vi "Update State on Cursor Move.vi"(8 "Cursor.Position.X":dbl, 9 "Cursor Name":string, 11 "Display State In":T1={"Graph Visible Items"={"Plot Legend"=FALSE, "Scale Legend"=FALSE, "Graph Palette"=FALSE, "Cursor Legend"=FALSE, "X Scrollbar"=FALSE}, "View Table"=FALSE, "Table Visible Items"={"Vertical Scrollbar"=FALSE, "Horizontal Scrollbar"=FALSE, "Row Headers"=FALSE, "Column Headers"=FALSE, "Vertical Lines"=FALSE, "Horizontal Lines"=FALSE}, "Header Font"={"Font Name"="", "Size"=0, "Bold"=FALSE, "Italic"=FALSE, "Underline"=FALSE, "Strikeout"=FALSE, "Color"=0}, "Cell Font"={"Font Name"="", "Size"=0, "Bold"=FALSE, "Italic"=FALSE, "Underline"=FALSE, "Strikeout"=FALSE, "Color"=0}, "Description and Tip..."={"Description"="", "Tip"=""}, "Moveable Splitter Position"=0, "Measurement Cursor Configuration"={"XY"={"enable XY"=FALSE, "Position (X)"=[], "Type"=enum."Absolute", "Y reference"=0.0, "color"=0}, "band"={"enable band"=FALSE, "B1"=0.0, "B2"=0.0, "Fixed bandwidth (B2-B1)"=0.0, "B1 color"=0, "B2 color"=0}, "harmonic"={"enable harmonics"=FALSE, "X reference (1X)"=0.0, "Maximum"=0, "Subset"=enum."All", "1X color"=0, "MX color"=0}, "sideband"={"enable sideband"=FALSE, "X center (C)"=0.0, "Sidebands"=0, "X spacing (s)"=0.0, "Center color"=0, "Sideband color"=0}}, "Cursors"={"List"=[], "Tags"=[]}, "X Increment"=0.0, "X Scale"={"Label Visible"=FALSE, "Label Text"="", "Mapping Mode"=0, "Format String"=""}, "Y Scale"={"Label Visible"=FALSE, "Label Text"="", "Mapping Mode"=0, "Format String"=""}, "Colors"={"background"=16777215, "major grid"=8355711, "minor grid"=12632256, "font"=0}, "desired spectrum view"={"scaling"={"linear/dB"=enum."no change", "dB reference"=0.0, "power/magnitude"=enum."no change", "view"=enum."no change"}, "spectral density"=enum."no change"}, "Plot Color Wheel"=[3381759, 32768, 982784, 4375295, 13827953, 13457919, 16757522, 4343295, 16728758, 12095254], "Plots"=[], "registered user events"=variant, "Lock 1X to Peak"=FALSE} caption="State" {"Y Scale"."Mapping Mode" items=["Linear", "Logarithmic", "dB"]; "X Scale"."Mapping Mode" items=["Linear", "Logarithmic"]}) -> (0 "cursor type":string, 1 "cursor index":i32, 3 "Display State Out":T1={"Graph Visible Items"={"Plot Legend"=FALSE, "Scale Legend"=FALSE, "Graph Palette"=FALSE, "Cursor Legend"=FALSE, "X Scrollbar"=FALSE}, "View Table"=FALSE, "Table Visible Items"={"Vertical Scrollbar"=FALSE, "Horizontal Scrollbar"=FALSE, "Row Headers"=FALSE, "Column Headers"=FALSE, "Vertical Lines"=FALSE, "Horizontal Lines"=FALSE}, "Header Font"={"Font Name"="", "Size"=0, "Bold"=FALSE, "Italic"=FALSE, "Underline"=FALSE, "Strikeout"=FALSE, "Color"=0}, "Cell Font"={"Font Name"="", "Size"=0, "Bold"=FALSE, "Italic"=FALSE, "Underline"=FALSE, "Strikeout"=FALSE, "Color"=0}, "Description and Tip..."={"Description"="", "Tip"=""}, "Moveable Splitter Position"=0, "Measurement Cursor Configuration"={"XY"={"enable XY"=FALSE, "Position (X)"=[], "Type"=enum."Absolute", "Y reference"=0.0, "color"=0}, "band"={"enable band"=FALSE, "B1"=0.0, "B2"=0.0, "Fixed bandwidth (B2-B1)"=0.0, "B1 color"=0, "B2 color"=0}, "harmonic"={"enable harmonics"=FALSE, "X reference (1X)"=0.0, "Maximum"=0, "Subset"=enum."All", "1X color"=0, "MX color"=0}, "sideband"={"enable sideband"=FALSE, "X center (C)"=0.0, "Sidebands"=0, "X spacing (s)"=0.0, "Center color"=0, "Sideband color"=0}}, "Cursors"={"List"=[], "Tags"=[]}, "X Increment"=0.0, "X Scale"={"Label Visible"=FALSE, "Label Text"="", "Mapping Mode"=0, "Format String"=""}, "Y Scale"={"Label Visible"=FALSE, "Label Text"="", "Mapping Mode"=0, "Format String"=""}, "Colors"={"background"=16777215, "major grid"=8355711, "minor grid"=12632256, "font"=0}, "desired spectrum view"={"scaling"={"linear/dB"=enum."no change", "dB reference"=0.0, "power/magnitude"=enum."no change", "view"=enum."no change"}, "spectral density"=enum."no change"}, "Plot Color Wheel"=[3381759, 32768, 982784, 4375295, 13827953, 13457919, 16757522, 4343295, 16728758, 12095254], "Plots"=[], "registered user events"=variant, "Lock 1X to Peak"=FALSE} caption="State" {"Y Scale"."Mapping Mode" items=["Linear", "Logarithmic", "dB"]; "X Scale"."Mapping Mode" items=["Linear", "Logarithmic"]})   [LabVIEW 2017, in "Octave with Cursors.xctl"]
doc: "Within Display State, moves linked cursors in set."
uses:
  <vilib>/addons/_XControls/Octave with Cursors/Octave with Cursors.xctl
  <vilib>/addons/_XControls/Octave with Cursors/Controls/State.ctl
  <vilib>/Utility/miscctls.llb/LVFontTypeDef.ctl
  <vilib>/addons/_XControls/Octave with Cursors/Controls/Measurement Cursor Configuration.ctl
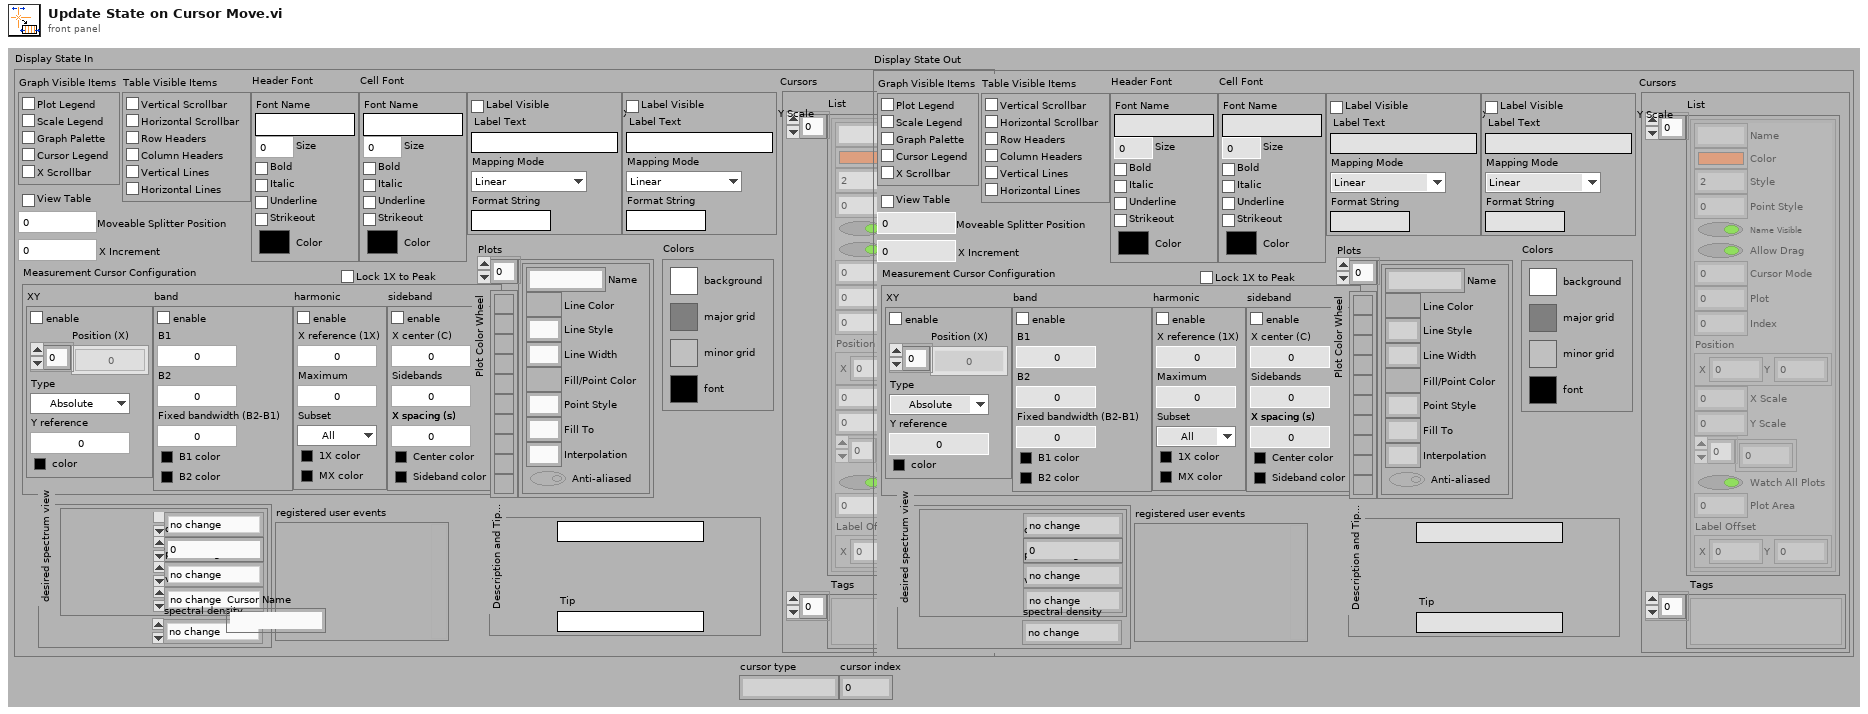
[diagram p1: front panel]
types:
  T1 = typedef "Octave with Cursors.xctl/State.ctl" = cluster{"Graph Visible Items":cluster{"Plot Legend":bool, "Scale Legend":bool, "Graph Palette":bool, "Cursor Legend":bool, "X Scrollbar":bool}, "View Table":bool, "Table Visible Items":cluster{"Vertical Scrollbar":bool, "Horizontal Scrollbar":bool, "Row Headers":bool, "Column Headers":bool, "Vertical Lines":bool, "Horizontal Lines":bool}, "Header Font":T2, "Cell Font":T2, "Description and Tip...":cluster{"Description":string, "Tip":string}, "Moveable Splitter Position":i32, "Measurement Cursor Configuration":T3, "Cursors":cluster{"List":cluster{"Name":string, "Color":u32, "Style":i32, "Point Style":u8, "Name Visible":bool, "Allow Drag":bool, "Cursor Mode":u32, "Plot":i32, "Index":i32, "Position":cluster{"X":dbl, "Y":dbl}, "X Scale":u32, "Y Scale":u32, "Watch Plots":i32[], "Watch All Plots":bool, "Plot Area":i32, "Label Offset":cluster{"X":dbl, "Y":dbl}}[], "Tags":variant[]}, "X Increment":dbl, "X Scale":cluster{"Label Visible":bool, "Label Text":string, "Mapping Mode":u8, "Format String":string}, "Y Scale":cluster{"Label Visible":bool, "Label Text":string, "Mapping Mode":u8, "Format String":string}, "Colors":cluster{"background":u32, "major grid":u32, "minor grid":u32, "font":u32}, "desired spectrum view":cluster{"scaling":cluster{"linear/dB":enum16{"no change", "linear", "dB"}, "dB reference":dbl, "power/magnitude":enum16{"no change", "power", "magnitude"}, "view":enum16{"no change", "rms", "peak", "peak-peak"}}, "spectral density":enum16{"no change", "spectrum", "spectral density"}}, "Plot Color Wheel":u32[], "Plots":cluster{"Name":string, "Line Color":u32, "Line Style":u8, "Line Width":u8, "Fill/Point Color":u32, "Point Style":u8, "Fill To":i16, "Interpolation":u8, "Anti-aliased":bool}[], "registered user events":variant, "Lock 1X to Peak":bool}
  T2 = typedef "LVFontTypeDef.ctl" = cluster{"Font Name":string, "Size":u16, "Bold":bool, "Italic":bool, "Underline":bool, "Strikeout":bool, "Color":u32}
  T3 = typedef "Octave with Cursors.xctl/Measurement Cursor Configuration.ctl" = cluster{"XY":cluster{"enable XY":bool, "Position (X)":dbl[], "Type":enum16{"Absolute", "Relative"}, "Y reference":dbl, "color":u32}, "band":cluster{"enable band":bool, "B1":dbl, "B2":dbl, "Fixed bandwidth (B2-B1)":dbl, "B1 color":u32, "B2 color":u32}, "harmonic":cluster{"enable harmonics":bool, "X reference (1X)":dbl, "Maximum":i32, "Subset":enum16{"All", "Even", "Odd"}, "1X color":u32, "MX color":u32}, "sideband":cluster{"enable sideband":bool, "X center (C)":dbl, "Sidebands":i32, "X spacing (s)":dbl, "Center color":u32, "Sideband color":u32}}
  T4 = cluster{"Name":string, "Color":u32, "Style":i32, "Point Style":u8, "Name Visible":bool, "Allow Drag":bool, "Cursor Mode":u32, "Plot":i32, "Index":i32, "Position":cluster{"X":dbl, "Y":dbl}, "X Scale":u32, "Y Scale":u32, "Watch Plots":i32[], "Watch All Plots":bool, "Plot Area":i32, "Label Offset":cluster{"X":dbl, "Y":dbl}}[]
  T5 = cluster{"Name":string, "Color":u32, "Style":i32, "Point Style":u8, "Name Visible":bool, "Allow Drag":bool, "Cursor Mode":u32, "Plot":i32, "Index":i32, "Position":cluster{"X":dbl, "Y":dbl}, "X Scale":u32, "Y Scale":u32, "Watch Plots":i32[], "Watch All Plots":bool, "Plot Area":i32, "Label Offset":cluster{"X":dbl, "Y":dbl}}
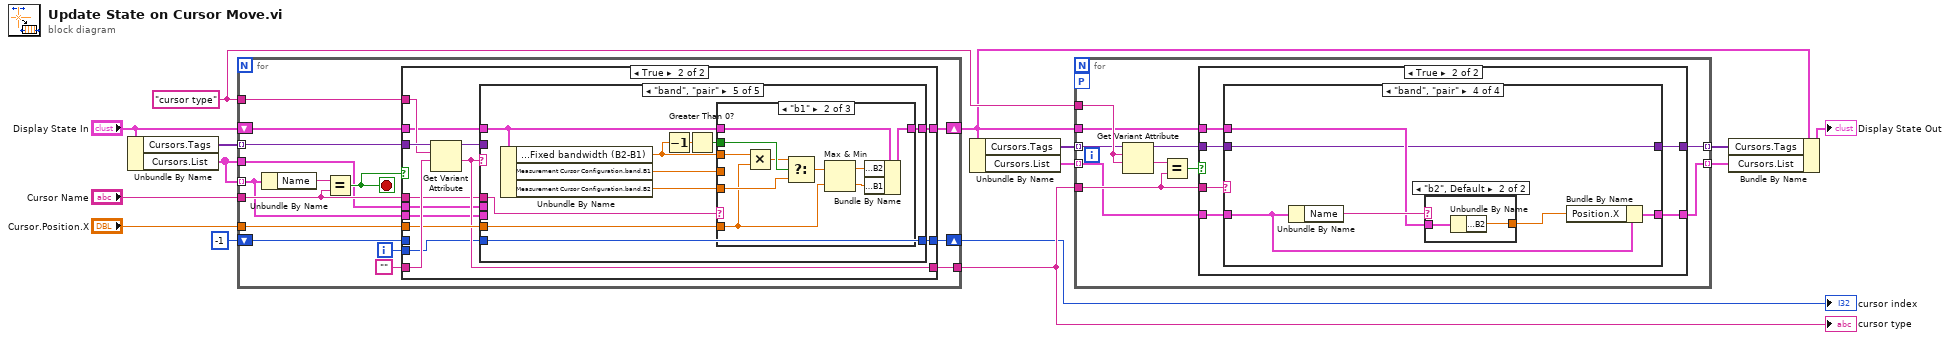
[diagram p0: block diagram]
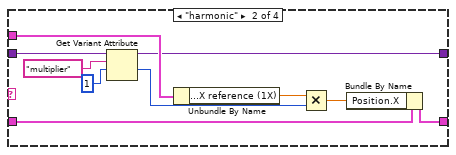
[diagram p4: hidden frame]
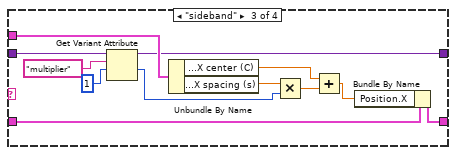
[diagram p5: hidden frame]
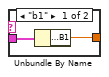
[diagram p6: hidden frame]
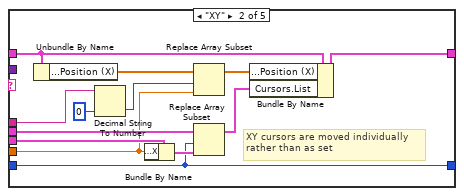
[diagram p9: hidden frame]
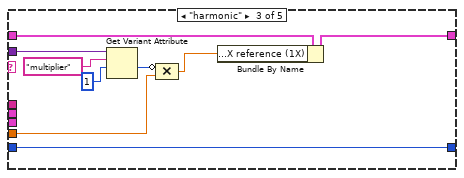
[diagram p10: hidden frame]
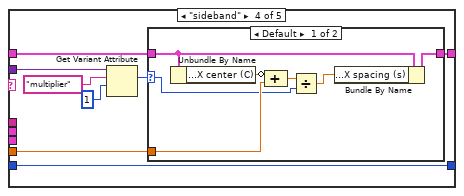
[diagram p11: hidden frame]
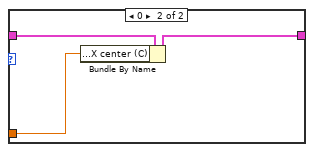
[diagram p12: hidden frame]
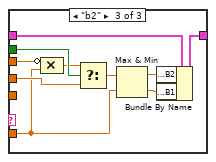
[diagram p14: hidden frame]
diagram:
  w15 = "cursor type"
  n1 = Unbundle By Name("Display State In") -> ("Cursors.Tags"=w10:variant[], "Cursors.List"=w5:T4)
  n2 = for {
    tunnel: "Cursor Name" -> [w26]
    tunnel: "Cursor.Position.X" -> [w27]
    shift-right: [w29] -> w3
    shift-left: "Display State In" -> [w30]
    tunnel: [w24] -> w4
    tunnel: w15 -> [w23]
    tunnel: w10 -> [w22] mode=indexing
    tunnel: w5 -> [w19] mode=indexing
    tunnel: w5 -> [w20]
    shift-right: [w18] -> w1
    shift-left: -1 -> [w16]
    i -> [w17]
    stop <- w25 stop-if-true
    n3 = Unbundle By Name(w19) -> ("Name"=w21:string)
    n4 = Equal?(x=w21, y=w26) -> (x = y?=w25:bool)
    n5 = case shown="True" w25 {
      tunnel: w22 -> [_ w46]
      tunnel: w23 -> [_ w45]
      tunnel: w30 -> [w33 w44]
      tunnel: [w33 w43] -> w29
      tunnel: w27 -> [_ w40]
      tunnel: w26 -> [_ w37]
      tunnel: [w32 w39] -> w24
      tunnel: w19 -> [_ w38]
      tunnel: w20 -> [_ w36]
      tunnel: "" -> [w32 w42]
      tunnel: w16 -> [w31 _]
      tunnel: [w31 w35] -> w18
      tunnel: w17 -> [_ w34]
      frame False {
      }
      frame True {
        n6 = Get Variant Attribute(Variant=w46, name=w45, default value (empty Variant)=w42) -> (duplicate Variant=w41:variant, value=w39:string)  [unwired: 1 in, 2 out]
        n7 = case shown="\"band\", \"pair\"" w39 {
          tunnel: w44 -> [w48 w59 w70 w78 w96]
          tunnel: [w48 w61 w69 w77 w98] -> w43
          tunnel: w41 -> [_ _ w68 w76 _]
          tunnel: w40 -> [_ w51 w65 w73 w97]
          tunnel: w37 -> [_ w55 _ _ w95]
          tunnel: w38 -> [_ w53 _ _ _]
          tunnel: w36 -> [_ w54 _ _ _]
          tunnel: w34 -> [w47 w49 w62 w71 w90]
          tunnel: [w47 w49 w62 w71 w90] -> w35
          frame Default {
          }
          frame "XY" {
            # "XY cursors are moved individually\nrather than as set"
            n8 = Unbundle By Name(w59) -> ("Measurement Cursor Configuration.XY.Position (X)"=w58:dbl[])
            n9 = Decimal String To Number(string=w55, default (0L)=0 ("default (0 I32)")) -> (number=w57:i32)  [unwired: 1 in, 1 out]
            n10 = Bundle By Name(cluster=w53, "Position.X"=w51) -> (w52:T5)
            n11 = Replace Array Subset(array=w58, new element=w51, index=w57) -> (w56:dbl[])
            n12 = Replace Array Subset(array=w54, new element=w52, index=w49) -> (w50:T4)
            n13 = Bundle By Name(cluster=w59, "Measurement Cursor Configuration.XY.Position (X)"=w56, "Cursors.List"=w50) -> (w61:T1)
          }
          frame "harmonic" {
            n14 = Get Variant Attribute(Variant=w68, name="multiplier", default value (empty Variant)=1) -> (value=w64:i32)  [unwired: 1 in, 3 out]
            n15 = Compound Arithmetic op=MULTIPLY(invert w64, w65) -> (w63:dbl)
            n16 = Bundle By Name(cluster=w70, "Measurement Cursor Configuration.harmonic.X reference (1X)"=w63) -> (w69:T1)
          }
          frame "sideband" {
            n17 = Get Variant Attribute(Variant=w76, name="multiplier", default value (empty Variant)=1) -> (value=w72:i32)  [unwired: 1 in, 3 out]
            n18 = case shown="Default" w72 {
              selector: w72 -> [w81 _]
              tunnel: w78 -> [w84 w88]
              tunnel: [w85 w87] -> w77
              tunnel: w73 -> [w82 w86]
              frame Default {
                n19 = Unbundle By Name(w84) -> ("Measurement Cursor Configuration.sideband.X center (C)"=w83:dbl)
                n20 = Compound Arithmetic op=ADD(invert w83, w82) -> (w80:dbl)
                n21 = Divide(x=w80, y=w81) -> (x/y=w79:dbl)
                n22 = Bundle By Name(cluster=w84, "Measurement Cursor Configuration.sideband.X spacing (s)"=w79) -> (w85:T1)
              }
              frame 0 {
                n23 = Bundle By Name(cluster=w88, "Measurement Cursor Configuration.sideband.X center (C)"=w86) -> (w87:T1)
              }
            }
          }
          frame "band", "pair" {
            n24 = Unbundle By Name(w96) -> ("Measurement Cursor Configuration.band.Fixed bandwidth (B2-B1)"=w91:dbl, "Measurement Cursor Configuration.band.B1"=w94:dbl, "Measurement Cursor Configuration.band.B2"=w93:dbl)
            n25 = Decrement(x=w91) -> (x-1=w89:dbl)
            n26 = Greater Than 0?(x=w89) -> (x > 0?=w92:bool)
            n27 = case shown="\"b1\"" w95 {
              tunnel: w96 -> [w99 w109 w119]
              tunnel: [w99 w108 w118] -> w98
              tunnel: w97 -> [_ w102 w110]
              tunnel: w94 -> [_ _ w111]
              tunnel: w93 -> [_ w104 _]
              tunnel: w91 -> [_ w106 w116]
              tunnel: w92 -> [_ w107 w117]
              frame Default {
              }
              frame "b1" {
                n28 = Multiply(x=w106, y=w102) -> (x*y=w105:dbl)
                n29 = Select(t=w105, s=w107, f=w104) -> (s? t:f=w103:dbl)
                n30 = Max & Min(x=w103, y=w102) -> (max(x,y)=w101:dbl, min(x,y)=w100:dbl)
                n31 = Bundle By Name(cluster=w109, "Measurement Cursor Configuration.band.B2"=w101, "Measurement Cursor Configuration.band.B1"=w100) -> (w108:T1)
              }
              frame "b2" {
                n32 = Compound Arithmetic op=MULTIPLY(invert w116, w110) -> (w115:dbl)
                n33 = Select(t=w115, s=w117, f=w111) -> (s? t:f=w114:dbl)
                n34 = Max & Min(x=w114, y=w110) -> (max(x,y)=w113:dbl, min(x,y)=w112:dbl)
                n35 = Bundle By Name(cluster=w119, "Measurement Cursor Configuration.band.B2"=w113, "Measurement Cursor Configuration.band.B1"=w112) -> (w118:T1)
              }
            }
          }
        }
      }
    }
  }
  "cursor type" <- w4
  "cursor index" <- w1
  n36 = Unbundle By Name(w3) -> ("Cursors.Tags"=w11:variant[], "Cursors.List"=w9:T4)
  n37 = for {
    tunnel: w11 -> [w124] mode=indexing
    tunnel: w15 -> [w129]
    tunnel: w4 -> [w125]
    tunnel: w9 -> [w123] mode=indexing
    tunnel: [w122] -> w8 mode=indexing
    tunnel: [w121] -> w6 mode=indexing
    tunnel: w3 -> [w120]
    workers-P: _ -> [_]
    n38 = Get Variant Attribute(Variant=w124, name=w129, default value (empty Variant)=w129) -> (duplicate Variant=w128:variant, value=w126:string)  [unwired: 1 in, 2 out]
    n39 = Equal?(x=w126, y=w125) -> (x = y?=w127:bool)
    n40 = case shown="True" w127 {
      tunnel: w128 -> [w131 w135]
      tunnel: w120 -> [_ w137]
      tunnel: w125 -> [_ w136]
      tunnel: w123 -> [w130 w134]
      tunnel: [w131 w133] -> w122
      tunnel: [w130 w132] -> w121
      frame False {
      }
      frame True {
        n41 = case shown="\"band\", \"pair\"" w136 {
          tunnel: w137 -> [_ w146 w161 w166]
          tunnel: w135 -> [w139 w149 w160 w165]
          tunnel: w134 -> [w138 w144 w153 w164]
          tunnel: [w139 w141 w150 w165] -> w133
          tunnel: [w138 w143 w152 w162] -> w132
          frame "XY", Default {
          }
          frame "harmonic" {
            n42 = Get Variant Attribute(Variant=w149, name="multiplier", default value (empty Variant)=1) -> (duplicate Variant=w141:variant, value=w140:i32)  [unwired: 1 in, 2 out]
            n43 = Unbundle By Name(w146) -> ("Measurement Cursor Configuration.harmonic.X reference (1X)"=w145:dbl)
            n44 = Multiply(x=w145, y=w140) -> (x*y=w142:dbl)
            n45 = Bundle By Name(cluster=w144, "Position.X"=w142) -> (w143:T5)
          }
          frame "sideband" {
            n46 = Get Variant Attribute(Variant=w160, name="multiplier", default value (empty Variant)=1) -> (duplicate Variant=w150:variant, value=w155:i32)  [unwired: 1 in, 2 out]
            n47 = Unbundle By Name(w161) -> ("Measurement Cursor Configuration.sideband.X center (C)"=w156:dbl, "Measurement Cursor Configuration.sideband.X spacing (s)"=w157:dbl)
            n48 = Multiply(x=w157, y=w155) -> (x*y=w154:dbl)
            n49 = Add(x=w156, y=w154) -> (x+y=w151:dbl)
            n50 = Bundle By Name(cluster=w153, "Position.X"=w151) -> (w152:T5)
          }
          frame "band", "pair" {
            n51 = Unbundle By Name(w164) -> ("Name"=w167:string)
            n52 = case shown="\"b2\", Default" w167 {
              tunnel: w166 -> [w169 w171]
              tunnel: [w168 w170] -> w163
              frame "b1" {
                n53 = Unbundle By Name(w169) -> ("Measurement Cursor Configuration.band.B1"=w168:dbl)
              }
              frame "b2", Default {
                n54 = Unbundle By Name(w171) -> ("Measurement Cursor Configuration.band.B2"=w170:dbl)
              }
            }
            n55 = Bundle By Name(cluster=w164, "Position.X"=w163) -> (w162:T5)
          }
        }
      }
    }
  }
  n56 = Bundle By Name(cluster=w3, "Cursors.Tags"=w8, "Cursors.List"=w6) -> (→"Display State Out":T1)
